vi "Crear Conexion.vi"(8 "error in (no error)":errorcluster, 11 "Serial Devices in":refnum<class "Serial Devices.lvclass">) -> (0 "error out":errorcluster, 3 "Serial Devices out":refnum<class "Serial Devices.lvclass">)   [LabVIEW 2019, in "Serial Devices.lvlib" / "Serial Devices.lvclass"]
uses:
  Serial Devices.lvclass
  Serial Devices.lvclass/Serial Devices.ctl
  NXP/NXP.lvclass
  TI/CYPRESS.lvclass
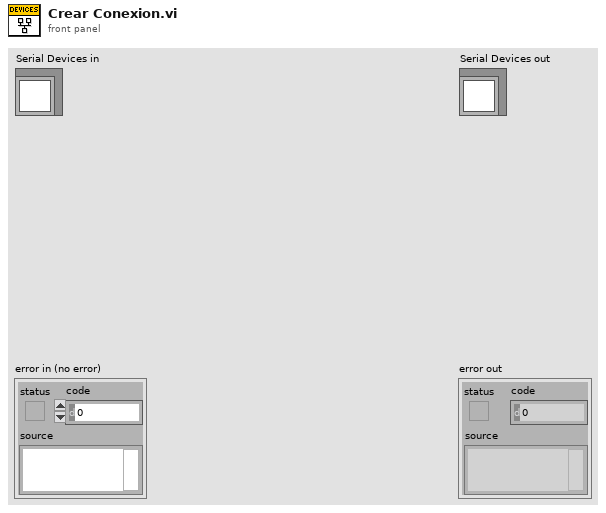
[diagram p1: front panel]
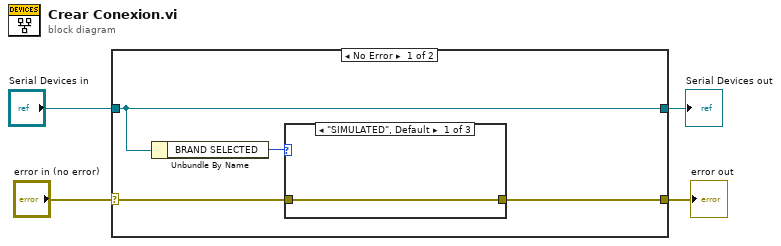
[diagram p0: block diagram]
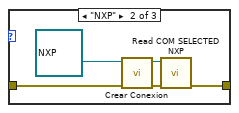
[diagram p2: hidden frame]
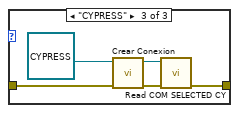
[diagram p3: hidden frame]
diagram:
  n1 = case shown="No Error" "error in (no error)" {
    selector: "error in (no error)" -> [w6 w21]
    tunnel: [w5 w21] -> w3
    tunnel: [w8 w20] -> w1
    tunnel: "Serial Devices in" -> [w8 w20]
    frame No Error {
      n2 = Unbundle By Name(w8) -> ("BRAND SELECTED"=w7:enum16{"NXP", "CYPRESS", "SIMULATED"})
      n3 = case shown="\"SIMULATED\", Default" w7 {
        tunnel: w6 -> [w9 w12 w18]
        tunnel: [w9 w10 w15] -> w5
        frame "SIMULATED", Default {
        }
        frame "NXP" {
          n4 = call-dynamic "Crear Conexion.vi"("error in (no error)"=w12, "NXP in"=refnum<class "NXP.lvclass"> refnum ("NXP.lvclass")) -> ("error out"=w11:errorcluster, "NXP out"=w13:refnum<class "NXP.lvclass">)  [unwired: 8 in]
          n5 = call "Read COM SELECTED NXP.vi"("error in (no error)"=w11, "NXP in"=w13) -> ("error out"=w10:errorcluster)  [unwired: 7 in, 2 out]
        }
        frame "CYPRESS" {
          n6 = call-dynamic "Crear Conexion.vi"("error in (no error)"=w18, "CYPRESS in"=refnum<class "CYPRESS.lvclass"> refnum ("CYPRESS.lvclass")) -> ("error out"=w16:errorcluster, "CYPRESS out"=w17:refnum<class "CYPRESS.lvclass">)  [unwired: 8 in]
          n7 = call "Read COM SELECTED CY.vi"("error in (no error)"=w16, "TI in"=w17) -> ("error out"=w15:errorcluster)  [unwired: 7 in, 2 out]
        }
      }
    }
    frame Error {
    }
  }
  "error out" <- w3
  "Serial Devices out" <- w1
